vi "G#RealTimeTemplate_CreateSub.vi"(0 "reference in":refnum<class "G#RealTimeTemplate.lvclass">, 5 "error in (no error)":errorcluster) -> (14 "reference out":refnum<class "G#RealTimeTemplate.lvclass">, 19 "error out":errorcluster)   [LabVIEW 2020, in "G#RealTimeTemplate.lvclass"]
doc: "Constructor."
uses:
  <vilib>/addons/_AddQ/G#Templates/G#RealTimeTemplate/G#RealTimeTemplate.lvclass
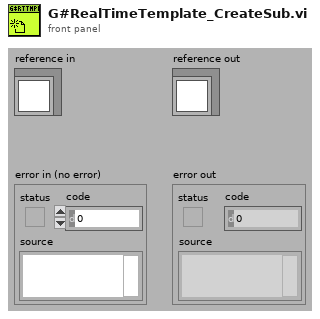
[diagram p1: front panel]
types:
  T1 = typedef "G#RealTimeTemplate.lvclass/ObjectAttributesRef.ctl" = refnum<data-value>
  T2 = typedef "G#RealTimeTemplate.lvclass/ObjectAttributes.ctl" = cluster{"MyAttribute":dbl}
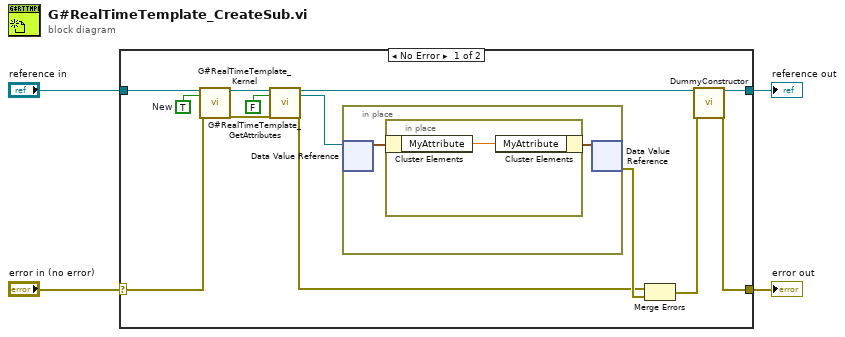
[diagram p0: block diagram]
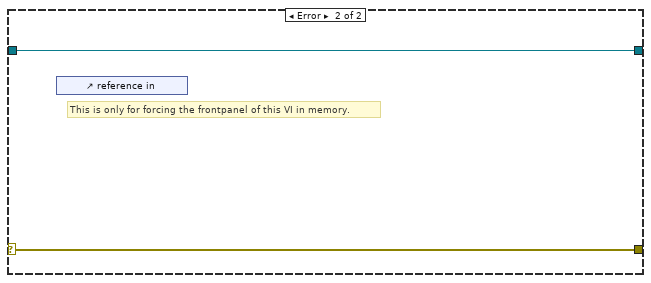
[diagram p2: hidden frame]
diagram:
  n1 = case shown="No Error" "error in (no error)" {
    selector: "error in (no error)" -> [w6 w22]
    tunnel: [w11 w22] -> w3
    tunnel: [w13 w21] -> w1
    tunnel: "reference in" -> [w8 w21]
    frame No Error {
      w9 = TRUE  # New
      n2 = call <vilib>:"G#RealTimeTemplate_Kernel.vi"("reference in"=w8, "New? (F=Dispose)"=w9, "error in (no error)"=w6) -> ("reference out"=w7:refnum<class "G#RealTimeTemplate.lvclass">, "error out"=w5:errorcluster)  [unwired: 15 in]
      n3 = call <vilib>:"G#RealTimeTemplate_GetAttributes.vi"("reference in"=w7, "return data? (T)"=FALSE, "error in (no error)"=w5) -> ("reference out"=w14:refnum<class "G#RealTimeTemplate.lvclass">, "attributes ref"=w16:T1, "error out"=w10:errorcluster)  [unwired: 13 in, 1 out]
      n4 = in-place {
        n5 = in-place-dvr #1(w16) -> (w18:T2)  [unwired: 1 out]
        n6 = in-place {
          n7 = in-place-cluster #2(w18) -> ("MyAttribute"=w20:dbl)
          n8 = in-place-cluster #2("MyAttribute"=w20) -> (w19:T2)
        }
        n9 = in-place-dvr #1(w19) -> (w17:errorcluster)  [unwired: 1 out]
      }
      n10 = Merge Errors(w10, w17) -> (w12:errorcluster)
      n11 = call <vilib>:"DummyConstructor.vi"("reference in"=w14, "error in (no error)"=w12) -> ("reference out"=w13:refnum<class "G#RealTimeTemplate.lvclass">, "error out"=w11:errorcluster)  [unwired: 16 in]
    }
    frame Error {
      # "This is only for forcing the frontpanel of this VI in memory."
      n12 = control-ref of="reference in"() -> ()  [unwired: 1 out]
    }
  }
  "error out" <- w3
  "reference out" <- w1
